vi "Init_DM_V2.vi"(7 "BM Flat":bool, 8 "BM Flat File":string, 9 "Mirror Modes File":string, 10 "DM Mapping File":string, 11 "Base File Path":path) -> (3 "reference out":refnum<k7>)   [LabVIEW 2014]
uses:
  <vilib>/Utility/file.llb/Read From Spreadsheet File (DBL).vi
  <vilib>/Analysis/Matrix/Numeric/Conversions/Array To Matrix - RA2.vi
  <vilib>/Utility/file.llb/Read From Spreadsheet File (string).vi
  <vilib>/Analysis/Matrix/NI_Matrix.lvlib
panel:
  out "IDs":i32[](array[numeric])
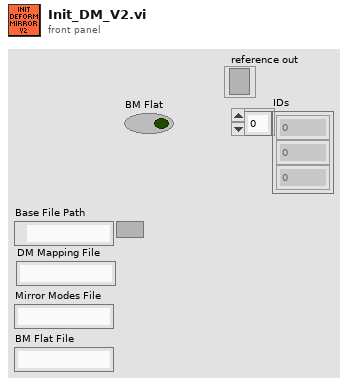
[diagram p1: front panel]
types:
  T1 = typedef "NI_Matrix.lvlib/RealMatrix.ctl" = dbl[][]
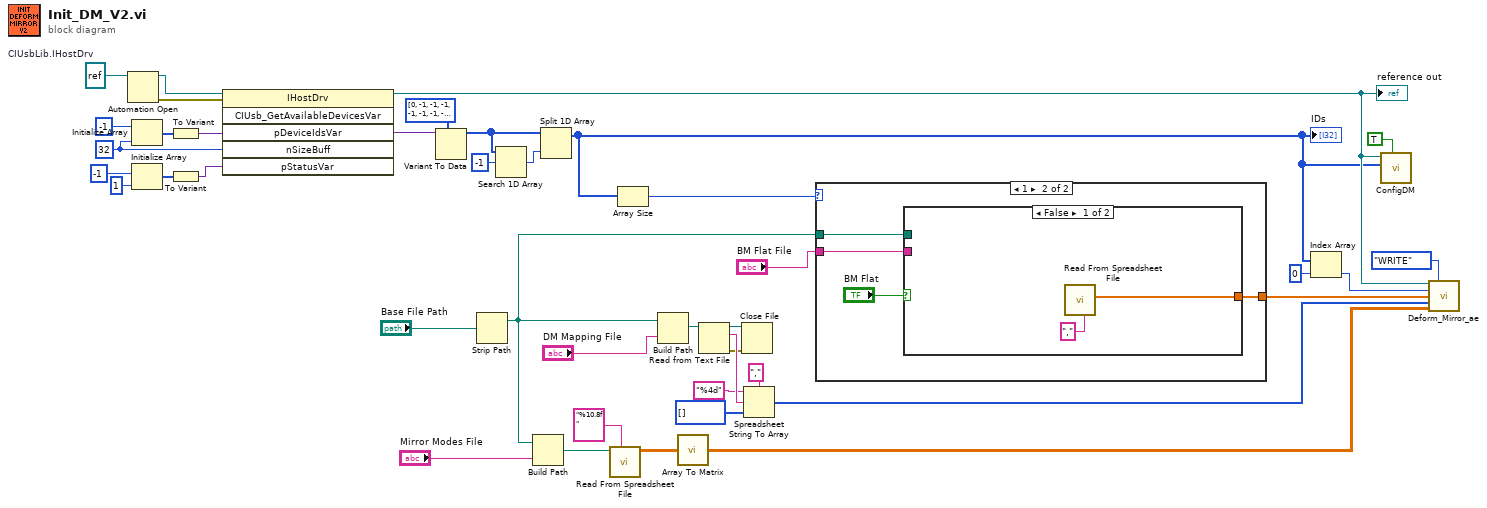
[diagram p0: block diagram]
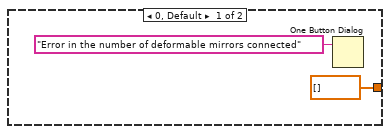
[diagram p2: hidden frame]
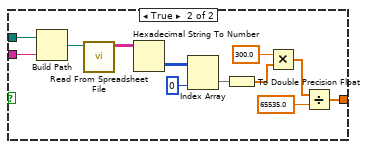
[diagram p3: hidden frame]
diagram:
  w36 = 32 ("dimension size")
  w27 = refnum<k7> refnum  # CIUsbLib.IHostDrv
  n1 = Automation Open(Automation Refnum=w27) -> (Automation Refnum=w32:refnum<k7>, error out=w33:errorcluster)  [unwired: 1 in, 2 out]
  n2 = Initialize Array(-1 ("element"), w36) -> (w29:i32[])
  n3 = Initialize Array(-1 ("element"), 1 ("dimension size")) -> (w28:i32[])
  n4 = To Variant(anything=w29) -> (Variant=w30:variant)
  n5 = To Variant(anything=w28) -> (Variant=w35:variant)
  n6 = invoke class="IHostDrv" method="CIUsb_GetAvailableDevicesVar"(reference=w32, error in=w33, "pDeviceIdsVar"=w30, "nSizeBuff"=w36, "pStatusVar"=w35) -> (reference out=w9:refnum<k7>, "pDeviceIdsVar"=w41:variant)  [unwired: 1 in, 4 out]
  "reference out" <- w9
  n7 = Variant To Data(type=i32[] [0, -1, -1, -1, -1, -1, -1, -1, -1, -1, -1, -1, -1, -1, -1, -1, -1, -1, -1, -1, -1, -1, -1, -1, -1, -1, -1, -1, -1, -1, -1, -1] ("pDeviceIDs"), Variant=w41) -> (data=w39:i32[])  [unwired: 1 in, 1 out]
  n8 = Strip Path(path="Base File Path") -> (stripped path=w17:path)  [unwired: 1 out]
  n9 = Search 1D Array(1D array=w39, element=-1) -> (index of element=w38:i32)  [unwired: 1 in]
  n10 = Build Path(base path=w17, name or relative path="Mirror Modes File") -> (appended path=w18:path)
  n11 = Split 1D Array(array=w39, index=w38) -> (first subarray=w8:i32[])  [unwired: 1 out]
  "IDs" <- w8
  n12 = call-poly <vilib>:"Read From Spreadsheet File.vi"("format (%.3f)"="%10.8f", "file path (dialog if empty)"=w18) -> ("all rows"=w7:dbl[][])  [unwired: 2 in, 7 out]
  n13 = Array Size(array=w8) -> (size(s)=w15:i32)
  n14 = Build Path(base path=w17, name or relative path="DM Mapping File") -> (appended path=w20:path)
  n15 = call-poly <vilib>:"Array To Matrix.vi"("Real 2D Array"=w7) -> ("Real Matrix"=w13:T1)
  n16 = Read from Text File(file (use dialog)=w20) -> (refnum out=w22:refnum<file>, text=w26:string, error out=w21:errorcluster)  [unwired: 1 in, 3 out]
  n17 = Close File(refnum=w22, error in=w21) -> ()  [unwired: 2 out]
  n18 = Spreadsheet String To Array(delimiter (Tab)=",", format string="%4d", spreadsheet string=w26, array type (2D Dbl)=i32[] []) -> (array=w11:i32[])
  n19 = case shown="1" w15 {
    tunnel: w17 -> [_ w47]
    tunnel: "BM Flat File" -> [_ w46]
    tunnel: [dbl[] [] w45] -> w14
    frame 0, Default {
      n20 = One Button Dialog(message="Error in the number of deformable mirrors connected") -> ()  [unwired: 1 in, 1 out]
    }
    frame 1 {
      n21 = case shown="False" "BM Flat" {
        tunnel: w47 -> [_ w61]
        tunnel: w46 -> [_ w60]
        tunnel: [w48 w51] -> w45
        frame False {
          n22 = call-poly <vilib>:"Read From Spreadsheet File.vi"("delimiter (\\t)"="," ("delimiter (\\t)")) -> ("first row"=w48:dbl[])  [unwired: 6 in, 4 out]
        }
        frame True {
          n23 = Build Path(base path=w61, name or relative path=w60) -> (appended path=w59:path)
          n24 = call-poly <vilib>:"Read From Spreadsheet File.vi"("file path (dialog if empty)"=w59) -> ("all rows"=w58:string[][])  [unwired: 3 in, 7 out]
          n25 = Hexadecimal String To Number(string=w58) -> (number=w57:u32[][])  [unwired: 2 in, 1 out]
          n26 = Index Array(array=w57, index (col)=0 ("disabled index (col)")) -> (element=w55:u32[])  [unwired: 1 in]
          n27 = To Double Precision Float(number=w55) -> (double precision float=w50:dbl[])
          n28 = Multiply(x=300.0 ("y"), y=w50) -> (x*y=w54:dbl[])
          n29 = Divide(x=w54, y=65535.0) -> (x/y=w51:dbl[])
        }
      }
    }
  }
  n30 = Index Array(array=w8, index=0) -> (element=w6:i32)
  n31 = call "ConfigDM.vi"("High Voltage"=TRUE, "Dev IDs"=w8, "Automation Refnum in"=w9) -> ()  [unwired: 7 in, 2 out]
  n32 = call "Deform_Mirror_ae.vi"("Refnum In"=w9, "Enum"=enum16{"WRITE", "READ"}."WRITE", "IDs In"=w6, "Flat Files In"=w14, "Multi Map Data In"=w11, "Mode Matrix In"=w13) -> ()  [unwired: 5 in, 5 out]
